vi "Kinesis - KSC101 - Set Operating Mode.vi"() -> ()   [LabVIEW 2012]
uses:
  U:/Kinesis LabVIEW Website Examples/Thorlabs.MotionControl.Controls.dll
  Thorlabs.MotionControl.Controls.dll
  U:/Kinesis LabVIEW Website Examples/Thorlabs.MotionControl.KCube.SolenoidCLI.dll
  Thorlabs.MotionControl.KCube.SolenoidCLI.dll
panel:
  in  "NumberOfCycles":i32
  in  "OpenTime":i32
  in  "ClosedTime":i32
  in  "?":bool
  in  "Serial Number":string
  in  "Start Shutter Sequence":bool
  in  "KCubeSolenoidControl":refnum<k24>(container)
  # "Notes:"
  # "- Ensure that the appropriate .DLLs are copied into your Project Folder. Check that the correct bit type are used depending on your version of LabVIEW\ni.e. 32-bit or 64-bit.\n\n\n\n\n\n\n\n\n\n\n\n\n\n\n- Open the example VI through the LabVIEW Project Explorer to correctly load the User Interface from Thorlabs.MotionControl.Controls.dll."
  # "Thorlabs Hardware: KSC101 - K-Cube Solenoid Controller\nhttps://www.thorlabs.com/newgrouppage9.cfm?objectgroup_id=2422\n\nThis VI will enable you to connect to a KSC101 Solenoid Controller, initialising the Kinesis UI panel. The VI will set the device in 'Auto' mode. In this mode, the solenoid will open and close continuously after the top panel wheel is moved up (primed). You are able to alter the settings of mode by using the 'SET OPERATING MODE' button. The progam will poll for updates to the 'SET OPERATING MODE' button controlling a case structure in the block diagram. If initiated the parameters of 'Auto' mode entered into the below controls will cause the device settings to be updated accordingly.\n\nInstructions:\n1) Connect your KSC101 device to your PC & power the device, ensuring your shutter device is connected. For full device setup, the device product manual can be found on our website here. - https://www.thorlabs.com/thorproduct.cfm?partnumber=KSC101\n2) Enter the device serial number below.\n3) Click 'Run' in the LabVIEW Toolbar to start the program.\n4) Assign values into the controls below. The range of values are detailed in the Kinesis .NET API - \nsee Thorlabs::MotionControl::KCube::SolenoidCLI::CycleSettings Class Reference."
  # "Example Image of .NET Controller - VI opened via Project Explorer/ not opened via Project Explorer"
  # "VI Not Opened via Project Explorer"
  # "VI Opened via Project Explorer"
  # "- To explore the range of methods available, please visit the .NET API, included with your Kinesis software.\n\n- For tips on building your own VIs with Thorlabs Motion Control Hardware, please see our LabVIEW Guide here.\nhttps://www.thorlabs.com/newgrouppage9.cfm?objectgroup_id=10285"
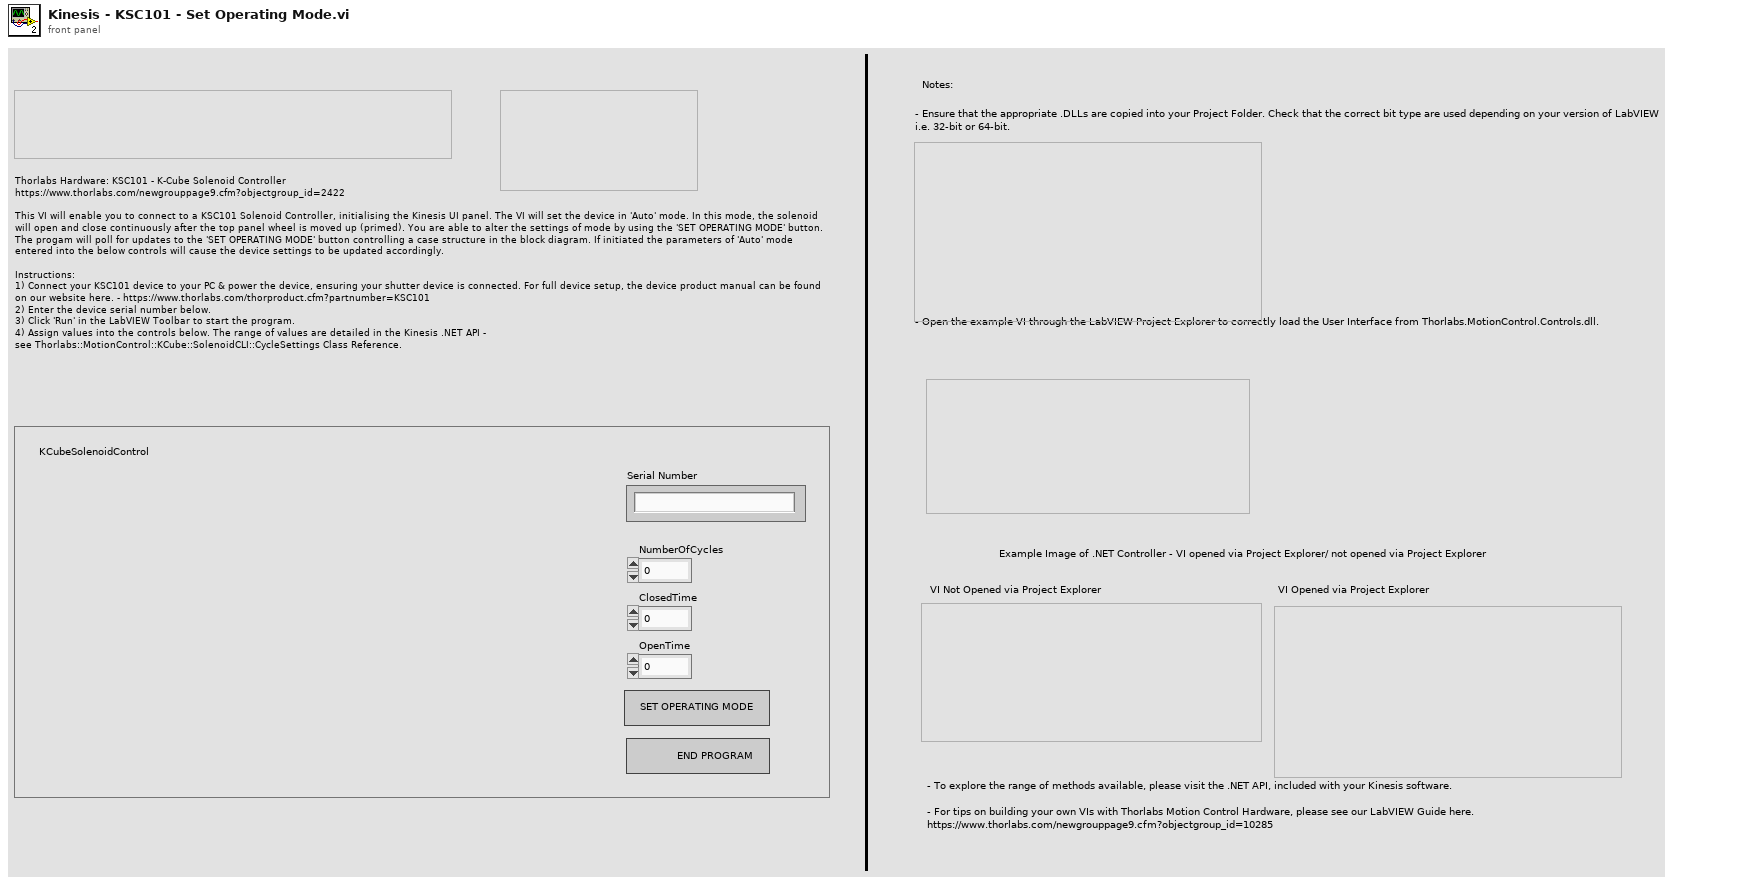
[diagram p1: front panel]
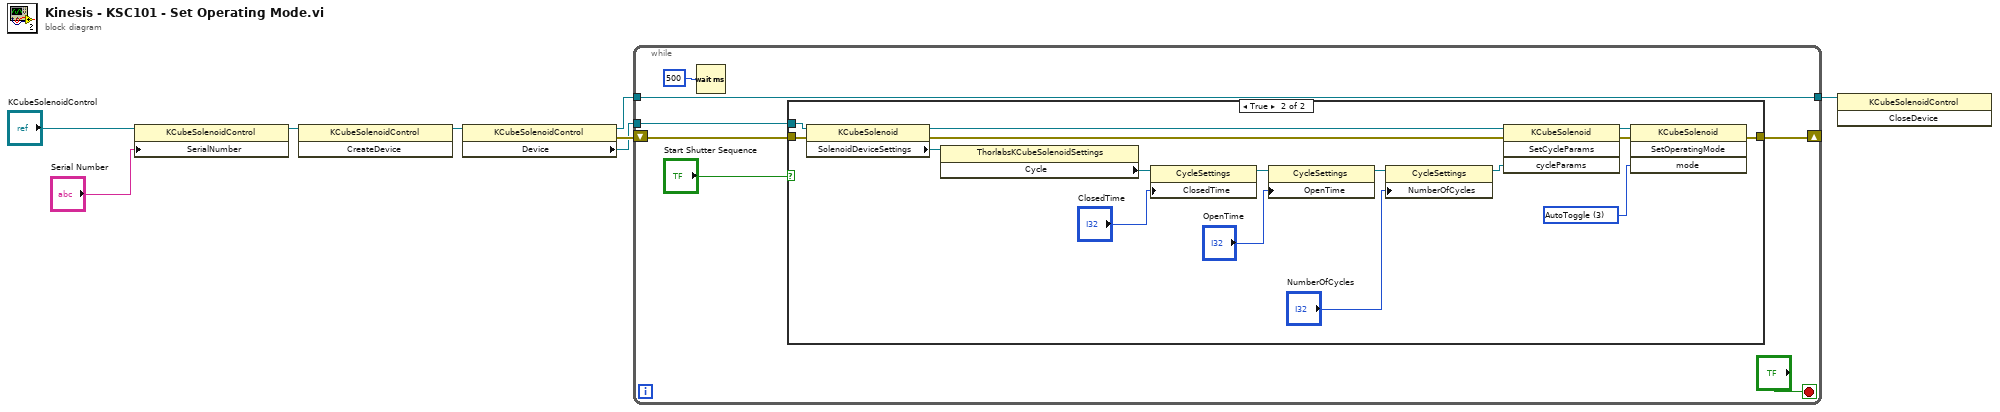
[diagram p0: block diagram]
diagram:
  n1 = property class="KCubeSolenoidControl"(reference="KCubeSolenoidControl", "SerialNumber"="Serial Number") -> (reference out=w4:refnum<k24>)  [unwired: 1 in, 1 out]
  n2 = invoke class="KCubeSolenoidControl" method="CreateDevice"(reference=w4) -> (reference out=w8:refnum<k24>)  [unwired: 2 in, 2 out]
  n3 = property class="KCubeSolenoidControl"(reference=w8) -> (reference out=w1:refnum<k24>, error out=w7:errorcluster, "Device"=w6:refnum<k24>)  [unwired: 1 in]
  n4 = while {
    tunnel: w6 -> [w15]
    shift-right: [w13] -> _
    shift-left: w7 -> [w14]
    tunnel: [w9] -> w2
    tunnel: w1 -> [w9]
    stop <- "?" stop-if-true
    n5 = Wait (ms)(milliseconds to wait=u32 500) -> ()  [unwired: 1 out]
    n6 = case shown="True" "Start Shutter Sequence" {
      tunnel: w15 -> [_ w30]
      tunnel: w14 -> [w16 w29]
      tunnel: [w16 w32] -> w13
      frame False {
      }
      frame True {
        w31 = 3 items=["Manual"=1, "SingleToggle"=2, "AutoToggle"=3, "Triggered"=4] ("mode")
        n7 = property class="KCubeSolenoid"(reference=w30, error in=w29) -> (reference out=w28:refnum<k24>, error out=w27:errorcluster, "SolenoidDeviceSettings"=w24:refnum<k24>)
        n8 = property class="ThorlabsKCubeSolenoidSettings"(reference=w24) -> ("Cycle"=w20:refnum<k24>)  [unwired: 1 in, 2 out]
        n9 = property class="CycleSettings"(reference=w20, "ClosedTime"="ClosedTime") -> (reference out=w23:refnum<k24>)  [unwired: 1 in, 1 out]
        n10 = property class="CycleSettings"(reference=w23, "OpenTime"="OpenTime") -> (reference out=w22:refnum<k24>)  [unwired: 1 in, 1 out]
        n11 = property class="CycleSettings"(reference=w22, "NumberOfCycles"="NumberOfCycles") -> (reference out=w21:refnum<k24>)  [unwired: 1 in, 1 out]
        n12 = invoke class="KCubeSolenoid" method="SetCycleParams"(reference=w28, error in=w27, "cycleParams"=w21) -> (reference out=w26:refnum<k24>, error out=w25:errorcluster)  [unwired: 1 in, 2 out]
        n13 = invoke class="KCubeSolenoid" method="SetOperatingMode"(reference=w26, error in=w25, "mode"=w31) -> (error out=w32:errorcluster)  [unwired: 1 in, 3 out]
      }
    }
  }
  n14 = invoke class="KCubeSolenoidControl" method="CloseDevice"(reference=w2) -> ()  [unwired: 2 in, 3 out]
